vi "Read Attributes.vi"(11 "Abstract Message Template in":refnum<class "Publish Camera Settings Msg.lvclass">) -> (2 "Payload":cluster{"Camera Settings":variant}, 3 "Abstract Message Template out":refnum<class "Publish Camera Settings Msg.lvclass">)   [LabVIEW 2020, in "Camera Actor.lvlib" / "Publish Camera Settings Msg.lvclass"]
uses:
  Publish Camera Settings Msg.lvclass
  Publish Camera Settings Msg.lvclass/Publish Camera Settings Msg.ctl
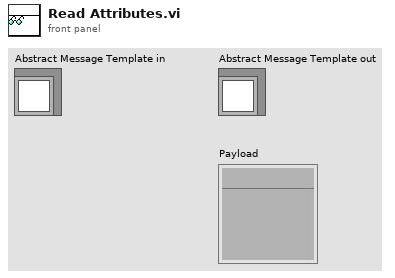
[diagram p1: front panel]
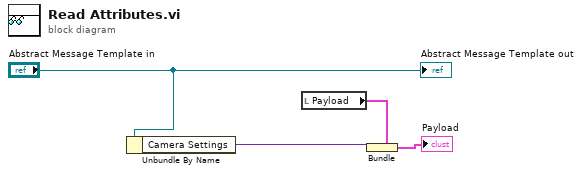
[diagram p0: block diagram]
diagram:
  n1 = Unbundle By Name("Abstract Message Template in") -> ("Camera Settings"=w1:variant)
  n2 = local read "Payload"() -> (w2:cluster{"Camera Settings":variant})
  n3 = Bundle(cluster=w2, "Camera Settings"=w1) -> (→"Payload":cluster{"Camera Settings":variant})
  "Abstract Message Template out" <- "Abstract Message Template in"
